vi "macro_vecBuilder8x1FIll.vi"   [LabVIEW 2019, in "Trajectory_Library.lvlib"]
uses:
  MatBuilder_Create.vi
  Trajectory_Library.lvlib
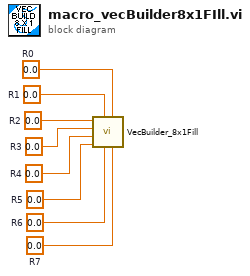
[diagram p0: block diagram]
diagram:
  w1 = 0.0  # R7
  w2 = 0.0  # R6
  w3 = 0.0  # R5
  w4 = 0.0  # R4
  w5 = 0.0  # R3
  w6 = 0.0  # R2
  w7 = 0.0  # R1
  w8 = 0.0  # R0
  n1 = call "VecBuilder_8x1Fill.vi"("R7"=w1, "R0"=w8, "R6"=w2, "R1"=w7, "R5"=w3, "R4"=w4, "R3"=w5, "R2"=w6) -> ()  [unwired: 3 in, 1 out]
